vi "Get Schedule Status.vi"(8 "error in (no error)":errorcluster, 11 "Monkey in":refnum<class "Monkey.lvclass">) -> (0 "error out":errorcluster, 1 "Empty?":bool, 2 "Schedule out":refnum<class "Schedule.lvclass">, 3 "Monkey out":refnum<class "Monkey.lvclass">)   [LabVIEW 2020, in "Monkey.lvlib" / "Monkey.lvclass"]
doc: "Returns the current Schedule and an indicator if it is empty or not"
uses:
  Monkey.lvclass
  Run Utilities/Schedule/Schedule.lvclass
  Run Utilities/Run Block/Run Block.lvclass
  Monkey.lvclass/Monkey.ctl
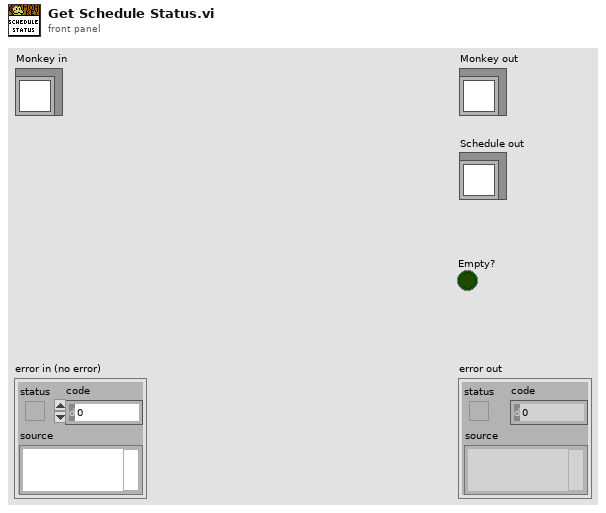
[diagram p1: front panel]
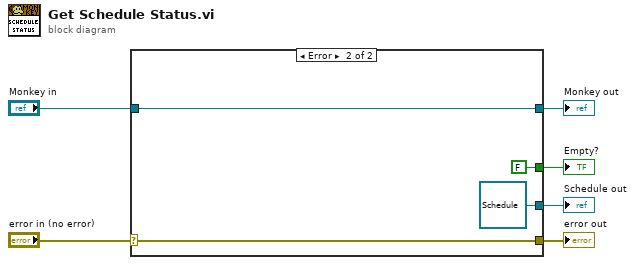
[diagram p0: block diagram]
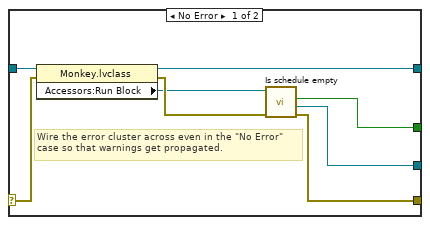
[diagram p2: hidden frame]
diagram:
  n1 = case shown="Error" "error in (no error)" {
    selector: "error in (no error)" -> [w11 w18]
    tunnel: [w10 w18] -> w5
    tunnel: [w12 w17] -> w3
    tunnel: "Monkey in" -> [w13 w17]
    tunnel: [w9 refnum<class "Schedule.lvclass"> refnum ("Schedule out")] -> w2
    tunnel: [w8 FALSE ("Empty?")] -> w1
    frame No Error {
      # "Wire the error cluster across even in the \"No Error\"\ncase so that warnings get propagated."
      n2 = property class="Monkey.lvclass"(reference=w13, error in=w11) -> (reference out=w12:refnum<class "Monkey.lvclass">, error out=w14:errorcluster, "Accessors:Run Block"=w7:refnum<class "Run Block.lvclass">)
      n3 = call-dynamic "Is schedule empty.vi"("error in (no error)"=w14, "Run Block in"=w7) -> ("error out"=w10:errorcluster, "Schedule out"=w9:refnum<class "Schedule.lvclass">, "Empty?"=w8:bool)  [unwired: 6 in, 1 out]
    }
    frame Error {
    }
  }
  "error out" <- w5
  "Monkey out" <- w3
  "Schedule out" <- w2
  "Empty?" <- w1
